vi "NameCheck.vi"(8 "error in (no error)":errorcluster, 10 "Name":string, 11 "VariableManagerRef in":refnum<vi>) -> (0 "error out":errorcluster, 1 "UsedAsSequenceIndex":bool, 2 "UsedAsVariable":bool, 3 "VariableManagerRef out":refnum<vi>)   [LabVIEW 2012, in "VariableManagerAPI.lvlib"]
doc: "Check the given Name agains database if it is used as a variable name or as a sequence index name (<B>idx</B>, <B>idx_f</B>, <B>idx_max</B>)."
uses:
  VariableManagerAPI.lvlib
  VariableManager/VariableManager.lvclass
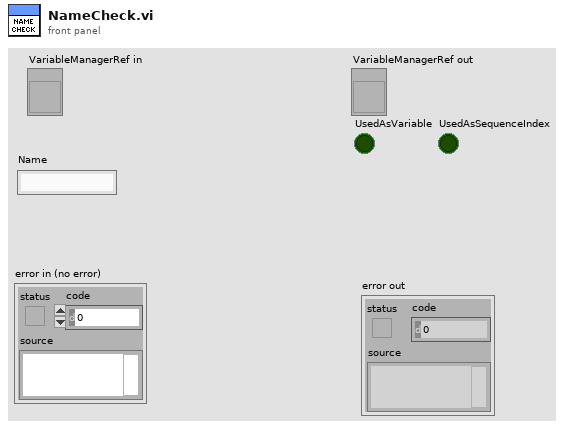
[diagram p1: front panel]
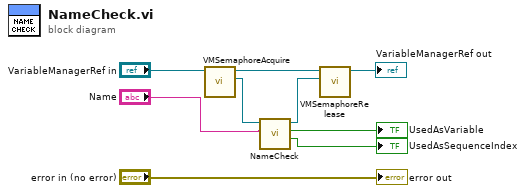
[diagram p0: block diagram]
diagram:
  n1 = call "VMSemaphoreAcquire.vi"("VariableManagerRef in"="VariableManagerRef in") -> ("VariableManager"=w5:refnum<class "VariableManager.lvclass">, "VariableManagerRef out"=w8:refnum<vi>)  [unwired: 7 in, 2 out]
  n2 = call-dynamic "NameCheck.vi"("Name"="Name", "VariableManager in"=w5) -> ("UsedAsSequenceIndex"=→"UsedAsSequenceIndex":bool, "UsedAsVariable"=→"UsedAsVariable":bool, "VariableManager out"=w1:refnum<class "VariableManager.lvclass">)  [unwired: 6 in, 1 out]
  n3 = call "VMSemaphoreRelease.vi"("VariableManager"=w1, "VariableManagerRef in"=w8) -> ("VariableManagerRef out"=→"VariableManagerRef out":refnum<vi>)  [unwired: 8 in, 1 out]
  "error out" <- "error in (no error)"
